vi "TSM SSC Digital Read Static.vi"(0 "Digital SSC in":T2, 11 "error in":errorcluster) -> (4 "Digital SSC out":T2, 6 "Per-Site Per-Pin data":T1[][](array[typedef]) items=["0"=0, "1"=1, "L"=3, "H"=4, "X"=5, "M"=6, "V"=7, "D"=8, "E"=9, "Not A Pin State"=254], 15 "error out":errorcluster)   [LabVIEW 2019]
doc: "Reads the current state of comparators for the specified pin(s) and pin group(s). If there are uncommitted changes to levels or the termination mode, this VI commits the changes to the pins. Returns an array of per-site per-pin static states."
uses:
  TSM/TSM SSC Digital.ctl
  <vilib>/NI_TestStand_SemiconductorModule/NI_TestStand_Semiconductor_Module.lvlibp/PinMap/Digital Pattern/PinQueryContext/DigitalPatternPinQueryContext.lvclass
  SSC Digital/SSC Digital.ctl
  <instrlib>/niDigital/niDigital.llb/niDigital Pin State.ctl
  03a3adb5-2161-439b-b621-88d6afab297a.vi
  Shared SubVIs/Channel List to Pins.vi
  Shared SubVIs/Trim Whitespace [Inlined].vi
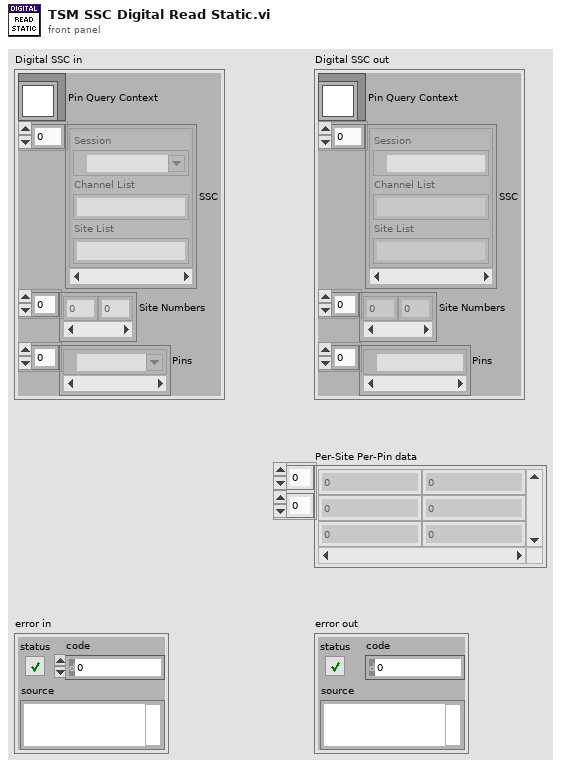
[diagram p1: front panel]
types:
  T1 = typedef "niDigital Pin State.ctl" = u8
  T2 = typedef "TSM SSC Digital.ctl" = cluster{"Pin Query Context":refnum<class "DigitalPatternPinQueryContext.lvclass">, "SSC":T3[], "Site Numbers":i32[], "Pins":tag[]}
  T3 = typedef "SSC Digital.ctl" = cluster{"Session":refnum<k15>, "Channel List":string, "Site List":string}
  T4 = typedef "Digital 2D Location Array in a Cluster.ctl" = cluster{"Digital 2D Location Array":T5[]}
  T5 = typedef "Digital 2D Location.ctl" = cluster{"Row":i32, "Col":i32}
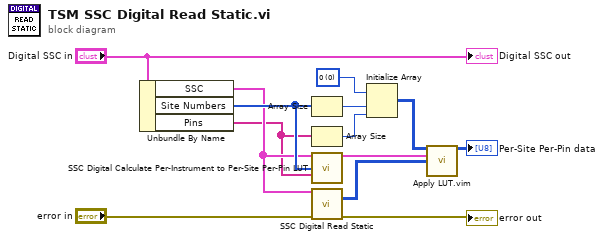
[diagram p0: block diagram]
diagram:
  w4 = T1 0 items=["0"=0, "1"=1, "L"=3, "H"=4, "X"=5, "M"=6, "V"=7, "D"=8, "E"=9, "Not A Pin State"=254] ("state")
  n1 = Unbundle By Name("Digital SSC in") -> ("SSC"=w7:T3[], "Site Numbers"=w8:i32[], "Pins"=w3:tag[])
  n2 = Array Size(array=w8) -> (size(s)=w10:i32)
  n3 = Array Size(array=w3) -> (size(s)=w2:i32)
  n4 = call "SSC Digital Calculate Per-Instrument to Per-Site Per-Pin LUT.vi"("Digital SSC In"=w7, "Sites"=w8, "Pins"=w3) -> ("Per-Instrument to Per-Site Per-Pin LUT"=w11:T4[])  [unwired: 12 in]
  n5 = call "SSC Digital Read Static.vi"("Digital SSC in"=w7, "error in"="error in") -> ("Per-Instrument Data"=w6:T1[][], "error out"=→"error out":errorcluster)  [unwired: 11 in, 1 out]
  n6 = Initialize Array(w4, w10, w2) -> (w9:T1[][])
  n7 = call "Apply LUT.vim"("Initialized Array"=w9, "LUT"=w11, "Results to Apply LUT to"=w6) -> ("Array Out"=→"Per-Site Per-Pin data":T1[][])  [unwired: 12 in]
  "Digital SSC out" <- "Digital SSC in"
